vi "求tv_start.vi"(3 "计算参数 in":T1, 5 "Array in":dbl[](array[numeric])) -> (0 "计算参数 out":T1, 2 "Array out":dbl[](array[numeric]))   [LabVIEW 2013]
doc: "搜索数组中第一个相邻元素差的绝对值大于0.01的元素，返回元素的索引"
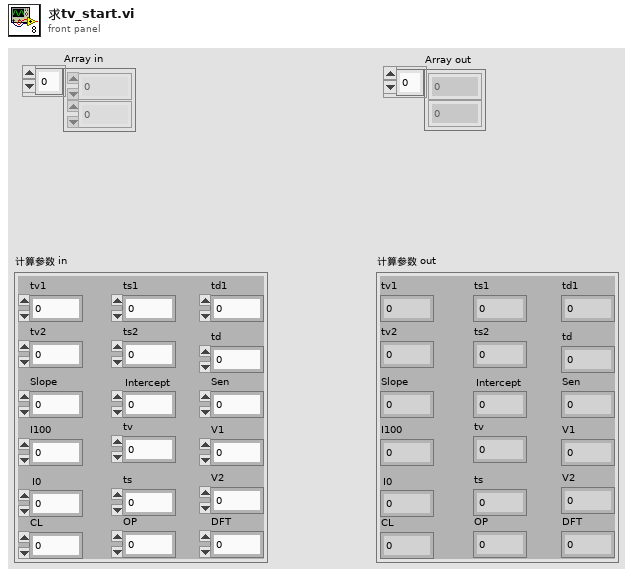
[diagram p1: front panel]
types:
  T1 = cluster{"tv1":dbl, "tv2":dbl, "tv":dbl, "ts1":dbl, "ts2":dbl, "ts":dbl, "td1":dbl, "td":dbl, "Slope":dbl, "Intercept":dbl, "I100":dbl, "I0":dbl, "Sen":dbl, "V1":dbl, "V2":dbl, "CL":dbl, "OP":dbl, "DFT":dbl}
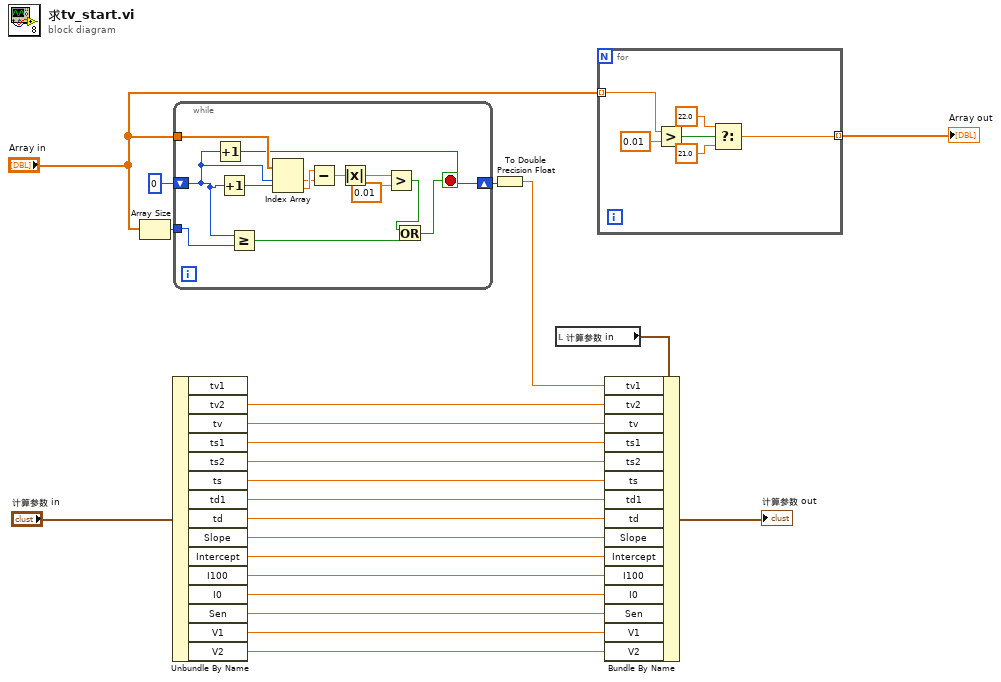
[diagram p0: block diagram]
diagram:
  n1 = Array Size(array="Array in") -> (size(s)=w21:i32)
  n2 = Unbundle By Name("计算参数 in") -> ("tv2"=w18:dbl, "tv"=w17:dbl, "ts1"=w16:dbl, "ts2"=w15:dbl, "ts"=w14:dbl, "td1"=w13:dbl, "td"=w12:dbl, "Slope"=w11:dbl, "Intercept"=w10:dbl, "I100"=w6:dbl, "I0"=w5:dbl, "Sen"=w9:dbl, "V1"=w8:dbl, "V2"=w7:dbl)  [unwired: 1 out]
  n3 = while {
    tunnel: "Array in" -> [w36]
    shift-right: [w30] -> w22
    shift-left: 0 -> [w25]
    tunnel: w21 -> [w29]
    stop <- w26 stop-if-true
    n4 = Increment(x=w25) -> (x+1=w30:i32)
    n5 = Increment(x=w25) -> (x+1=w24:i32)
    n6 = Greater Or Equal?(x=w25, y=w29) -> (x >= y?=w28:bool)
    n7 = Index Array(array=w36, index #1=w25, index #2=w24) -> (element #1=w34:dbl, element #2=w35:dbl)
    n8 = Subtract(x=w35, y=w34) -> (x-y=w33:dbl)
    n9 = Absolute Value(x=w33) -> (abs(x)=w32:dbl)
    n10 = Greater?(x=w32, y=0.01) -> (0:w27:bool)
    n11 = Or(x=w27, y=w28) -> (x .or. y?=w26:bool)
  }
  n12 = To Double Precision Float(number=w22) -> (double precision float=w3:dbl)
  n13 = local read "计算参数 in"() -> (w4:T1)
  n14 = for {
    tunnel: "Array in" -> [w41] mode=indexing
    tunnel: [w37] -> w1 mode=indexing
    n15 = Greater?(x=w41, y=0.01) -> (0:w40:bool)
    n16 = Select(t=22.0, s=w40, f=21.0) -> (s? t:f=w37:dbl)
  }
  "Array out" <- w1
  n17 = Bundle By Name(cluster=w4, "tv1"=w3, "tv2"=w18, "tv"=w17, "ts1"=w16, "ts2"=w15, "ts"=w14, "td1"=w13, "td"=w12, "Slope"=w11, "Intercept"=w10, "I100"=w6, "I0"=w5, "Sen"=w9, "V1"=w8, "V2"=w7) -> (→"计算参数 out":T1)
